vi "NISE.remote.Open Generic Property.vi"(0 "SLSC Remote in":refnum<class "SLSC Interface.lvclass">, 5 "resource":string, 7 "property in":refnum<k21>, 11 "error in (no error)":errorcluster) -> (4 "SLSC Remote out":refnum<class "SLSC Interface.lvclass">, 8 "property out":refnum<k21>, 15 "error out":errorcluster)   [LabVIEW 2016, in "SLSC Interface.lvclass"]
uses:
  SLSC Interface Class/SLSC Interface.lvclass
  SLSC Interface Class/SLSC Interface.lvclass/SLSC Interface.ctl
  SLSC Interface Class/NISE.Read client handle.vi
  SLSC Interface Class/NISE.Read URL.vi
  <vilib>/NI/JSON Support for LabVIEW/JSON Data Classes/JSON Object/JSON Object.lvclass
  C:/Program Files (x86)/National Instruments/LabVIEW 2016/vi.lib/NI/JSON Support for LabVIEW/JSON Data Classes/JSON Datatype/JSON Null.lvclass
  SLSC Interface Class/NISE.Read session.vi
  <vilib>/NI/JSON Support for LabVIEW/JSON Data Classes/JSON Object/New JSON Object (Empty).vi
  <vilib>/NI/JSON Support for LabVIEW/JSON Data Classes/JSON Object/Insert Key Value Pair (Single String).vi
  <vilib>/NI/NI JSONRPC Server Framework/Classes/Server/Format Client Request (Auto-Increment).vi
  <vilib>/httpClient/POSTBuffer.vi
  <vilib>/NI/NI JSONRPC Server Framework/Classes/Server/Parse Response (Object).vi
  <vilib>/NI/NI JSONRPC Server Framework/Classes/Server/JSONRPC Server.lvclass
  <vilib>/httpClient/LabVIEWHTTPClient.lvlib
  <vilib>/NI/JSON Support for LabVIEW/JSON Data Classes/JSON Helper/JSON Helper.lvclass
  C:/Program Files (x86)/National Instruments/LabVIEW 2016/vi.lib/NI/JSON Support for LabVIEW/JSON Data Classes/JSON Structured Type/JSON Structure.lvclass
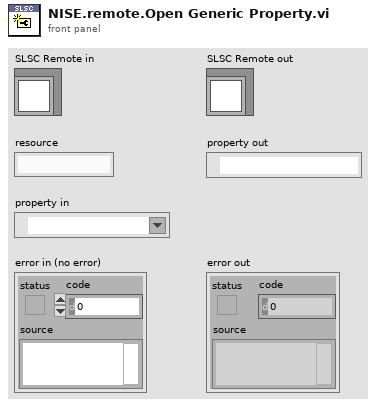
[diagram p1: front panel]
types:
  T1 = typedef "LabVIEWHTTPClient.lvlib/ClientHandle.ctl" = refnum<k1>
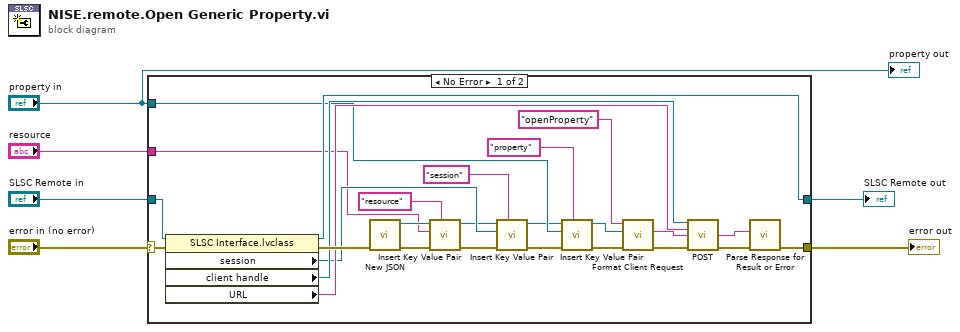
[diagram p0: block diagram]
diagram:
  n1 = case shown="No Error" "error in (no error)" {
    selector: "error in (no error)" -> [w30 w33]
    tunnel: "property in" -> [w15 _]
    tunnel: "SLSC Remote in" -> [w32 w34]
    tunnel: [w31 w34] -> w5
    tunnel: [w22 w33] -> w3
    tunnel: "resource" -> [w8 _]
    frame No Error {
      n2 = property class="SLSC Interface.lvclass"(reference=w32, error in=w30) -> (reference out=w31:refnum<class "SLSC Interface.lvclass">, error out=w29:errorcluster, "session"=w12:refnum<k21>, "client handle"=w27:T1, "URL"=w26:string)
      n3 = call-poly <vilib>:"New JSON.vi"("error in (no error)"=w29) -> ("error out"=w17:errorcluster, "JSON Object out"=w9:refnum<class "JSON Object.lvclass">)  [unwired: 9 in]
      n4 = call-poly <vilib>:"Insert Key Value Pair.vi"("key"="resource" ("Name"), "error in (no error)"=w17, "value"=w8, "JSON Object in"=w9) -> ("error out"=w16:errorcluster, "JSON Object out"=w11:refnum<class "JSON Object.lvclass">)  [unwired: 5 in, 1 out]
      n5 = call-poly <vilib>:"Insert Key Value Pair.vi"("key"="session" ("Name"), "error in (no error)"=w16, "value"=w12, "JSON Object in"=w11) -> ("error out"=w21:errorcluster, "JSON Object out"=w13:refnum<class "JSON Object.lvclass">)  [unwired: 5 in, 1 out]
      n6 = call-poly <vilib>:"Insert Key Value Pair.vi"("key"="property" ("Name"), "error in (no error)"=w21, "value"=w15, "JSON Object in"=w13) -> ("error out"=w19:errorcluster, "JSON Object out"=w20:refnum<class "JSON Object.lvclass">)  [unwired: 5 in, 1 out]
      n7 = call-poly <vilib>:"Format Client Request.vi"("error in (no error)"=w19, "JSON in"=w20, "method"="openProperty") -> ("error out"=w25:errorcluster, "Request String"=w28:string)  [unwired: 7 in]
      n8 = call-poly <vilib>:"POST.vi"("client handle"=w27, "url"=w26, "buffer"=w28, "error in (no error)"=w25) -> ("body"=w24:string, "error out"=w23:errorcluster)  [unwired: 8 in, 2 out]
      n9 = call-poly <vilib>:"Parse Response for Result or Error.vi"("error in"=w23, "Response String In"=w24) -> ("error out"=w22:errorcluster)  [unwired: 7 in, 2 out]
    }
    frame Error {
    }
  }
  "error out" <- w3
  "SLSC Remote out" <- w5
  "property out" <- "property in"
